vi "How to play.vi"() -> ()   [LabVIEW 2019]
panel:
  in  "Close Button":bool
  out "String":string
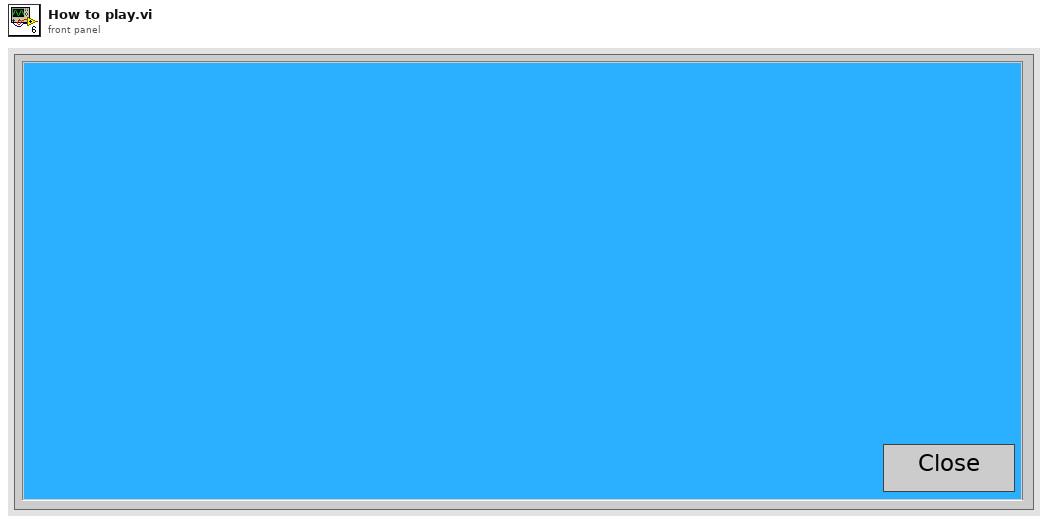
[diagram p1: front panel]
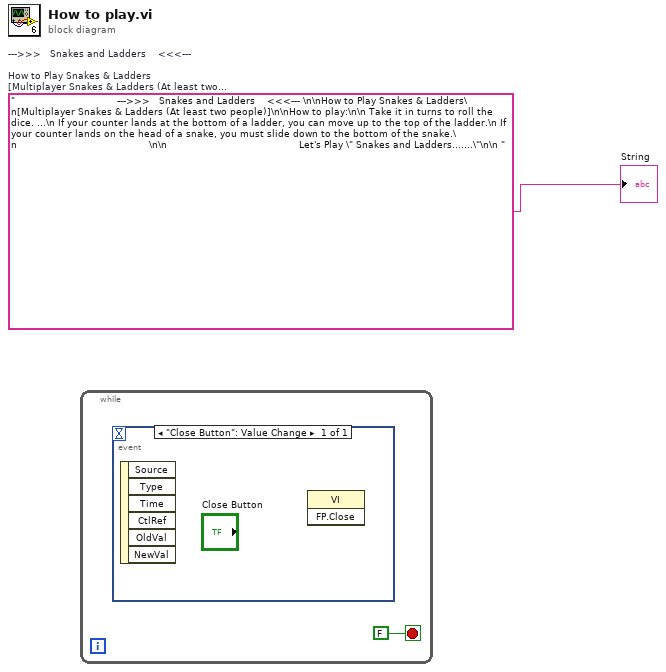
[diagram p0: block diagram]
diagram:
  w1 = "                                  --->>>   Snakes and Ladders    <<<--- \n\nHow to Play Snakes & Ladders\n[Multiplayer Snakes & Ladders (At least two people)]\n\nHow to play:\n\n Take it in turns to roll the dice. ...\n If your counter lands at the bottom of a ladder, you can move up to the top of the ladder.\n If your counter lands on the head of a snake, you must slide down to the bottom of the snake.\n                                            \n\n                                            Let's Play \" Snakes and Ladders.......\"\n\n "  # --->>>   Snakes and Ladders    <<<---   How to Play Snakes & Ladders [Multiplayer Snakes & Ladders (At least two people)]  How to play:   Take it in turns to roll the dice. ...  If your counter lands at the bottom of a ladder, you can move up to the top of the ladder.  If your counter lands on the head of a snake, you must slide down to the bottom of the snake.                                                                                           Let's Play " Snakes and Ladders......."
  n1 = while {
    stop <- FALSE stop-if-true
    n2 = event shown="[0] \"Close Button\": Value Change" {
      selector: _ -> [_]
      dyn-events: _ -> [_]
      timeout: _ -> [_]
      event "Close Button": Value Change {
        n3 = event-data() -> ()  [unwired: 1 in, 6 out]
        n4 = invoke class="VI" method="FP.Close"() -> ()  [unwired: 3 in, 3 out]
      }
    }
  }
  "String" <- w1
